vi "Calculate Required Steering Angle.vi"(7 "constraint error tolerance (1E-12)":dbl=1e-12, 8 "error in (no error)":errorcluster, 9 "wheel frame velocity":dbl[](array[numeric]), 11 "wheel in":refnum<class "NI_Robotics_Wheel.lvclass">) -> (0 "error out":errorcluster, 2 "required steering angle (rad)":dbl, 3 "wheel out":refnum<class "NI_Robotics_Wheel.lvclass">)   [LabVIEW 2017, in "NI_Robotics_Wheel.lvclass"]
uses:
  <vilib>/robotics/Steering/Wheel/NI_Robotics_Wheel.lvclass
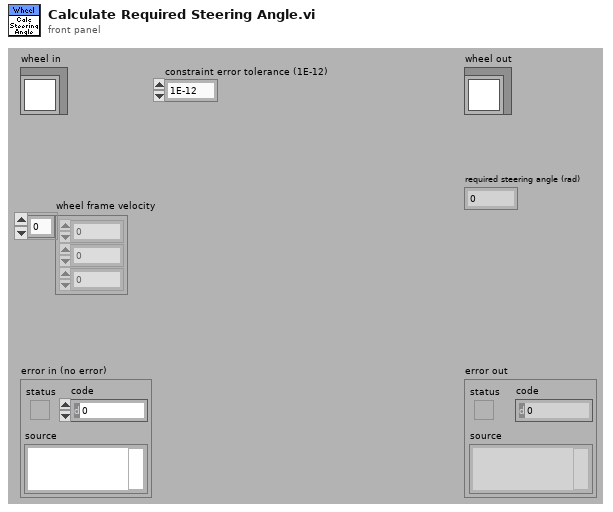
[diagram p1: front panel]
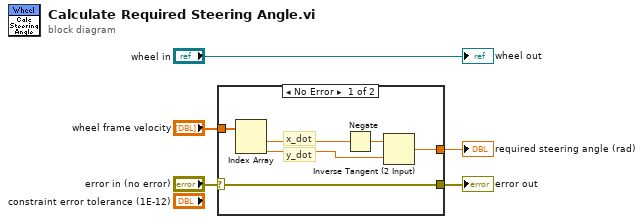
[diagram p0: block diagram]
diagram:
  n1 = case shown="No Error" "error in (no error)" {
    selector: "error in (no error)" -> [w10 w12]
    tunnel: "wheel frame velocity" -> [w11 _]
    tunnel: [w6 _] -> w3
    tunnel: [w10 w12] -> w1
    frame No Error {
      # "y_dot"
      # "x_dot"
      n2 = Index Array(array=w11) -> (element #1=w9:dbl, element #2=w7:dbl)  [unwired: 2 in]
      n3 = Negate(x=w9) -> (-x=w8:dbl)
      n4 = Inverse Tangent (2 Input)(1:w7, 2:w8) -> (0:w6:dbl)
    }
    frame Error {
    }
  }
  "error out" <- w1
  "required steering angle (rad)" <- w3
  "wheel out" <- "wheel in"
